vi "Globals.vi"() -> ()   [LabVIEW 2017, in "nifxpmath_Reciprocal.xnode"]
uses:
  <vilib>/rvi/FXPMathLib/FxpReciprocal/XNode/nifxpmath_Reciprocal.xnode
panel:
  out "SMALL ICON w/ 4WIRE":picture
  out "MIN WORD LENGTH":i32=1
  in  "TERM 1/X NAME":string="1/x"
  in  "TERM X NAME":string="x"
  in  "TERM OVFL ID":string="TERM_OVFL"
  in  "TERM 1/X ID":string="TERM_1/X"
  in  "TERM X ID":string="TERM_X"
  out "SMALL ICON":picture
  out "NORMAL BANNER":picture
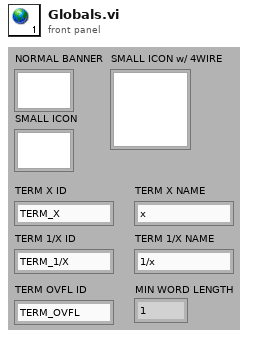
[diagram p1: front panel]
diagram:
